vi "b-fields many sensors one orbit point.vi"(6 "t0":fxp<+,48,48>, 8 "omega":dbl format="%#_13g", 9 "L":dbl, 10 "magnetometer readings":T3, 11 "orbit parameters":T2) -> (1 "measured field":dbl[](array[numeric]), 2 "derivatives":dbl[][](array[numeric]), 3 "predicted field":dbl[](array[numeric]), 4 "predicted location":dbl[](array[numeric]), 5 "sensor0 prediction":dbl[](array[numeric]), 7 "sensor0 measured":dbl[](array[numeric]))   [LabVIEW 2017]
uses:
  typedefs/magnetomter reading set.ctl
  typedefs/orbit parameters full.ctl
  typedefs/magnet location tx ty.ctl
  <vilib>/Analysis/baseanly.llb/Real A x B.vi
  <vilib>/Analysis/Matrix/Numeric/Conversions/Array To Matrix - RA2.vi
  <vilib>/Analysis/Matrix/Numeric/Conversions/Matrix To Array - RM.vi
  <vilib>/Analysis/Matrix/NI_Matrix.lvlib
  <vilib>/Analysis/NI_AALBase.lvlib
panel:
  out "magnet location tx ty BrV":T1
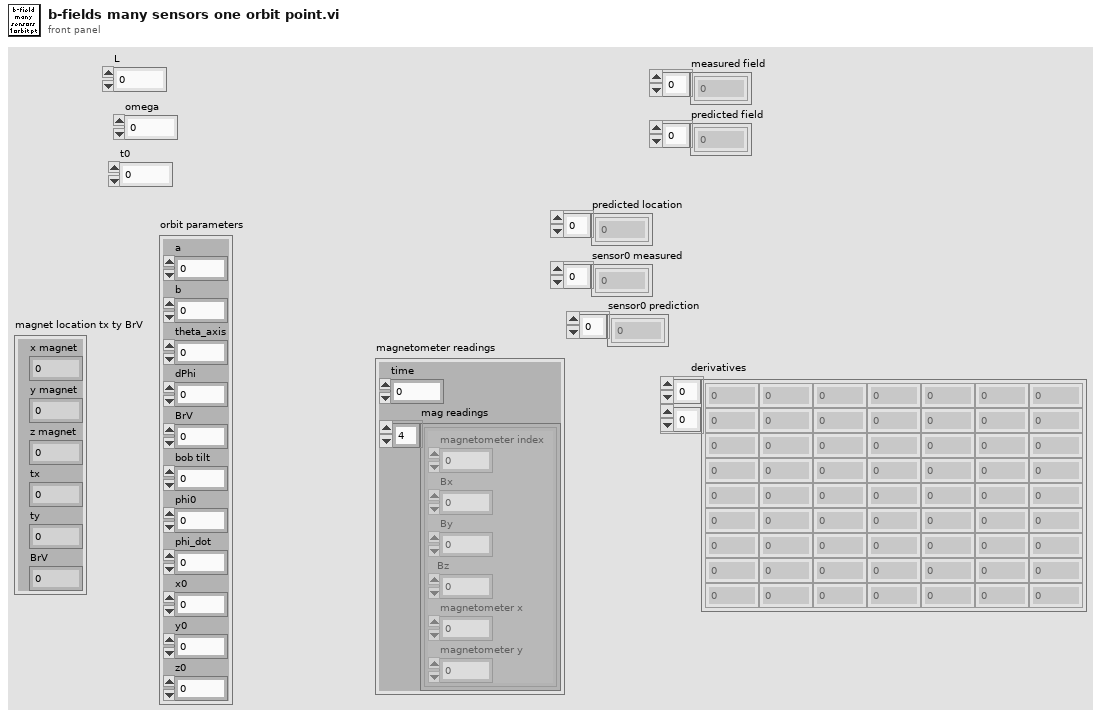
[diagram p1: front panel]
types:
  T1 = typedef "magnet location tx ty.ctl" = cluster{"x magnet":dbl, "y magnet":dbl, "z magnet":dbl, "tx":dbl, "ty":dbl, "BrV":dbl}
  T2 = typedef "orbit parameters full.ctl" = cluster{"a":dbl, "b":dbl, "theta_axis":dbl, "dPhi":dbl, "BrV":dbl, "bob tilt":dbl, "phi0":dbl, "phi_dot":dbl, "x0":dbl, "y0":dbl, "z0":dbl}
  T3 = typedef "magnetomter reading set.ctl" = cluster{"time":fxp<+,48,48>, "mag readings":cluster{"magnetometer index":dbl, "Bx":dbl, "By":dbl, "Bz":dbl, "magnetometer x":dbl, "magnetometer y":dbl}[]}
  T4 = cluster{"[0]":dbl, "[1]":dbl, "[2]":dbl, "[3]":dbl, "[4]":dbl, "[5]":dbl}
  T5 = typedef "NI_Matrix.lvlib/RealMatrix.ctl" = dbl[][]
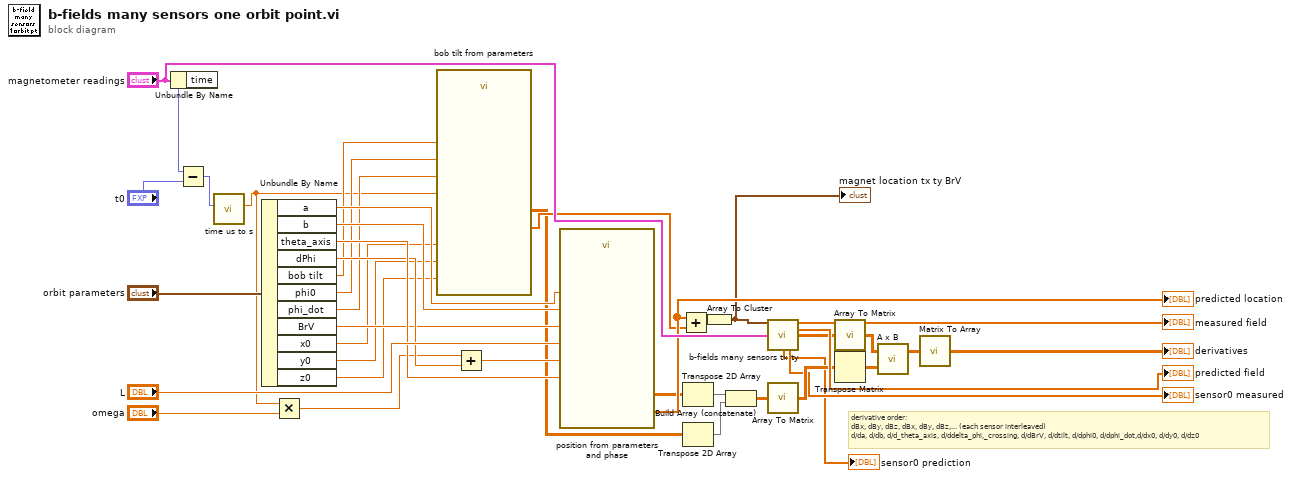
[diagram p0: block diagram]
diagram:
  # "derivative order:\ndBx, dBy, dBz, dBx, dBy, dBz,... (each sensor interleaved)\nd/da, d/db, d/d_theta_axis, d/ddelta_phi,_crossing, d/dBrV, d/dtilt, d/dphi0, d/dphi_dot,d/dx0, d/dy0, d/dz0"
  n1 = Unbundle By Name("magnetometer readings") -> ("time"=w26:fxp<+,48,48>)
  n2 = Subtract(x=w26, y="t0") -> (x-y=w2:fxp<+/-,49,49>)
  n3 = call "time us to s.vi"("time (us)"=w2) -> ("time (s)"=w1:dbl)  [unwired: 10 in]
  n4 = Unbundle By Name("orbit parameters") -> ("a"=w34:dbl, "b"=w33:dbl, "theta_axis"=w32:dbl, "dPhi"=w31:dbl, "bob tilt"=w30:dbl, "phi0"=w29:dbl, "phi_dot"=w28:dbl, "BrV"=w27:dbl, "x0"=w8:dbl, "y0"=w7:dbl, "z0"=w6:dbl)
  n5 = Multiply(x=w1, y="omega") -> (x*y=w24:dbl)
  n6 = call "bob tilt from parameters.vi"("y0"=w7, "z0"=w6, "x0"=w8, "t"=w1, "phi_dot"=w28, "phi0"=w29, "bob tilt"=w30) -> ("derivatives (i,j) = dOut(i) / dParam(j)"=w18:dbl[][], "Out = (x,y,z,tx,ty,BrV)"=w21:dbl[])  [unwired: 3 in]
  n7 = Add(x=w24, y=w31) -> (x+y=w23:dbl)
  n8 = call "position from parameters and phase.vi"("L"="L", "BrV"=w27, "phase"=w23, "theta_axis"=w32, "b"=w33, "a"=w34) -> ("derivatives (i,j) = dOut(i) / dParam(j)"=w19:dbl[][], "Out = (x,y,z,tx,ty)"=w22:dbl[])  [unwired: 4 in]
  "predicted location" <- w22
  n9 = Add(x=w22, y=w21) -> (x+y=w20:dbl[])
  n10 = Transpose 2D Array(2D array=w19) -> (transposed array=w17:dbl[][])
  n11 = Transpose 2D Array(2D array=w18) -> (transposed array=w15:dbl[][])
  n12 = Array To Cluster(array=w20) -> (cluster=w3:T4)
  "magnet location tx ty BrV" <- w3
  n13 = Build Array (concatenate)(w17, w15) -> (w16:dbl[][])
  n14 = call "b-fields many sensors tx ty.vi"("magnet location tx ty BrV"=w3, "Magnetometer reading set"="magnetometer readings") -> ("mf - flat"=→"measured field":dbl[], "pf - flat"=→"predicted field":dbl[], "derivative"=w13:dbl[][], "sensor0 prediction"=→"sensor0 prediction":dbl[], "sensor0 measured"=→"sensor0 measured":dbl[])  [unwired: 9 in]
  n15 = call-poly <vilib>:"Array To Matrix.vi"("Real 2D Array"=w16) -> ("Real Matrix"=w11:T5)
  n16 = call-poly <vilib>:"Array To Matrix.vi"("Real 2D Array"=w13) -> ("Real Matrix"=w14:T5)
  n17 = Transpose Matrix(1:w11) -> (0:w10:T5)
  n18 = call-poly <vilib>:"A x B.vi"("B"=w10, "A"=w14) -> ("A x B"=w12:T5)  [unwired: 1 out]
  n19 = call-poly <vilib>:"Matrix To Array.vi"("Real Matrix"=w12) -> ("Real 2D Array"=→"derivatives":dbl[][])
